vi "Cache.DUT.DataToTable.vi"(10 "Groups":i32[](array[numeric]), 11 "Results in":T1[](array[typedef])) -> (1 "Colors":u32[][](array[colorbox]), 2 "Headers":string[](array[string]), 3 "Values":string[][](array[string]))   [LabVIEW 2016]
uses:
  Database/Database.Global.vi
  Database/ProdaNG/Controls/ProdaNG.ProcessResult.ctl
  Database/ProdaNG/Controls/ProdaNG.ProcessStepResult.ctl
  Database/ProdaNG/Controls/ProdaNG.TestValueResult.ctl
  Database/ProdaNG/Controls/ProdaNG.TestStepResult.ctl
  Cache.TestSteps.Fglb.ResultData.ctl
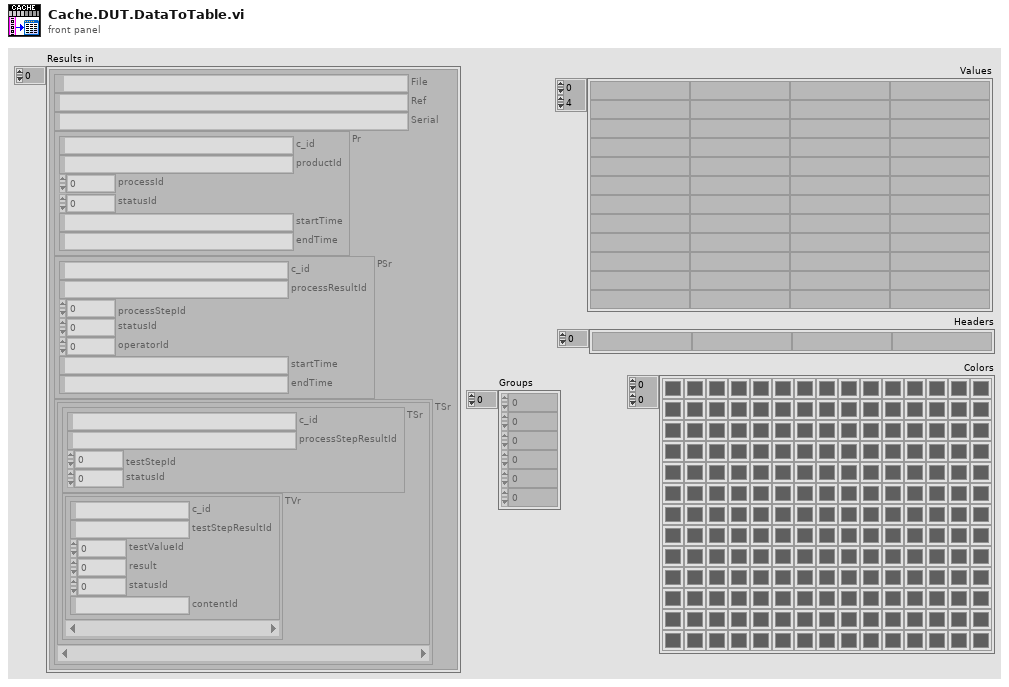
[diagram p1: front panel]
types:
  T1 = typedef "Cache.TestSteps.Fglb.ResultData.ctl" = cluster{"File":path, "Ref":string, "Serial":string, "Pr":T2, "PSr":T3, "TSr":cluster{"TSr":T4, "TVr":T5[]}[]}
  T2 = typedef "ProdaNG.ProcessResult.ctl" = cluster{"c_id":string, "productId":string, "processId":i32, "statusId":i32, "startTime":string, "endTime":string}
  T3 = typedef "ProdaNG.ProcessStepResult.ctl" = cluster{"c_id":string, "processResultId":string, "processStepId":i32, "statusId":i32, "operatorId":i32, "startTime":string, "endTime":string}
  T4 = typedef "ProdaNG.TestStepResult.ctl" = cluster{"c_id":string, "processStepResultId":string, "testStepId":i32, "statusId":i32}
  T5 = typedef "ProdaNG.TestValueResult.ctl" = cluster{"c_id":string, "testStepResultId":string, "testValueId":i32, "result":dbl, "statusId":i32, "contentId":string}
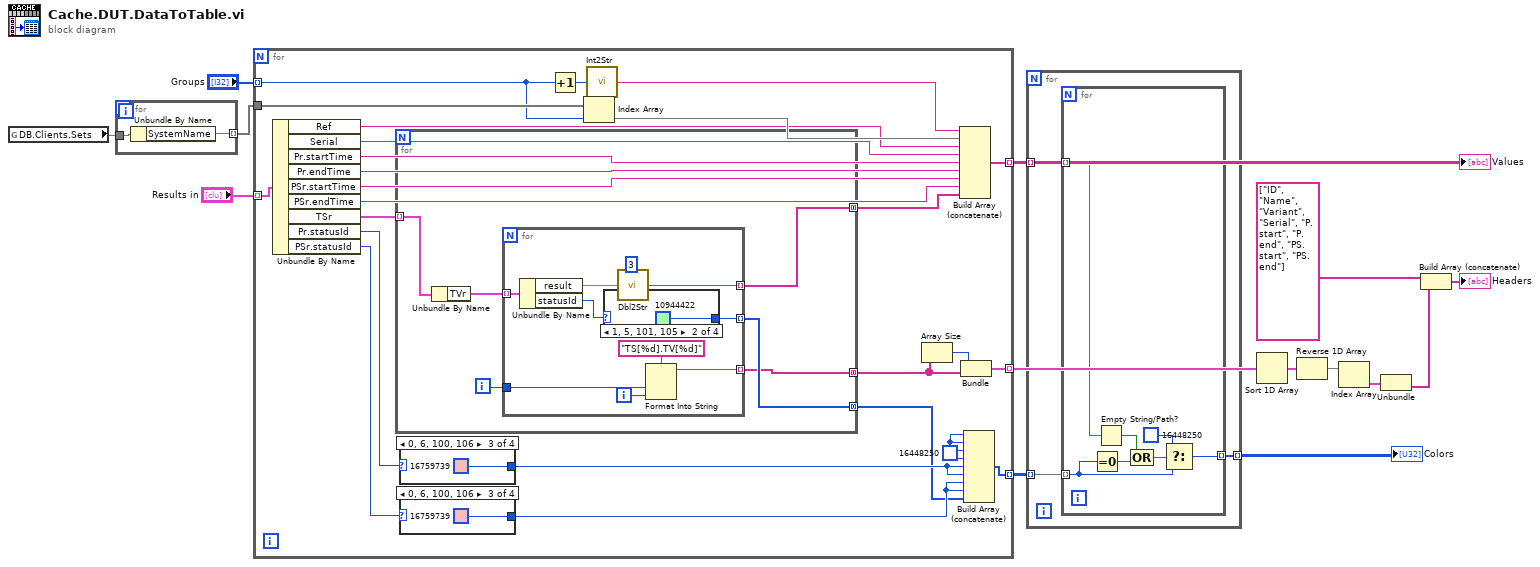
[diagram p0: block diagram]
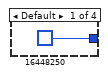
[diagram p2: hidden frame]
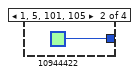
[diagram p3: hidden frame]
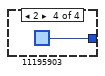
[diagram p4: hidden frame]
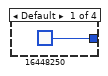
[diagram p5: hidden frame]
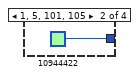
[diagram p6: hidden frame]
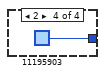
[diagram p7: hidden frame]
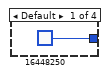
[diagram p8: hidden frame]
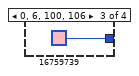
[diagram p9: hidden frame]
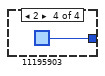
[diagram p10: hidden frame]
diagram:
  n1 = global read "Database.Global.vi" "DB.Clients.Sets"() -> (w10)
  n2 = for {
    tunnel: w10 -> [w16]
    tunnel: [w15] -> w1 mode=indexing
    n3 = Unbundle By Name(w16) -> ("SystemName"=w15)
  }
  n4 = for {
    tunnel: "Results in" -> [w41] mode=indexing
    tunnel: [w31] -> w12 mode=indexing
    tunnel: [w30] -> w13 mode=indexing
    tunnel: "Groups" -> [w21] mode=indexing
    tunnel: w1 -> [w27]
    tunnel: [w23] -> w9 mode=indexing
    w17 = u32 16448250
    n5 = Unbundle By Name(w41) -> ("Ref"=w19:string, "Serial"=w20:string, "Pr.startTime"=w40:string, "Pr.endTime"=w26:string, "PSr.startTime"=w39:string, "PSr.endTime"=w18:string, "TSr"=w38:cluster{"TSr":T4, "TVr":T5[]}[], "Pr.statusId"=w37:i32, "PSr.statusId"=w36:i32)
    n6 = for {
      tunnel: w38 -> [w55] mode=indexing
      tunnel: [w52] -> w33 mode=concatenating
      tunnel: [w51] -> w32 mode=concatenating
      tunnel: [w50] -> w24 mode=concatenating
      i -> [w53]
      n7 = Unbundle By Name(w55) -> ("TVr"=w54:T5[])
      n8 = for {
        tunnel: w54 -> [w65] mode=indexing
        tunnel: [w61] -> w52 mode=indexing
        tunnel: [w60] -> w51 mode=indexing
        tunnel: w53 -> [w57]
        tunnel: [w56] -> w50 mode=indexing
        i -> [w59]
        n9 = Unbundle By Name(w65) -> ("result"=w63:dbl, "statusId"=w64:i32)
        n10 = case shown="1, 5, 101, 105" w64 {
          tunnel: [u32 16448250 u32 10944422 u32 16759739 u32 11195903] -> w61
          frame Default {
          }
          frame 1, 5, 101, 105 {
          }
          frame 0, 6, 100, 106 {
          }
          frame 2 {
          }
        }
        n11 = call "Dbl2Str.vi"("Numeric"=w63, "precision (6)"=i16 3) -> ("string"=w60:string)
        n12 = Format Into String(format string="TS[%d].TV[%d]", w57, w59) -> (resulting string=w56:string)  [unwired: 2 in, 1 out]
      }
    }
    n13 = case shown="0, 6, 100, 106" w37 {
      tunnel: [u32 16448250 u32 10944422 u32 16759739 u32 11195903] -> w34
      frame Default {
      }
      frame 1, 5, 101, 105 {
      }
      frame 0, 6, 100, 106 {
      }
      frame 2 {
      }
    }
    n14 = case shown="0, 6, 100, 106" w36 {
      tunnel: [u32 16448250 u32 10944422 u32 16759739 u32 11195903] -> w35
      frame Default {
      }
      frame 1, 5, 101, 105 {
      }
      frame 0, 6, 100, 106 {
      }
      frame 2 {
      }
    }
    n15 = Increment(x=w21) -> (x+1=w28:i32)
    n16 = Index Array(array=w27, index=w21) -> (element=w25)
    n17 = call "Int2Str.vi"("Numeric"=w28) -> ("string"=w29:string)
    n18 = Array Size(array=w24) -> (size(s)=w22:i32)
    n19 = Build Array (concatenate)(w29, w25, w19, w20, w40, w26, w39, w18, w32) -> (w31:string[])
    n20 = Bundle(w22, w24) -> (w23:cluster{i32, string[]})  [unwired: 1 in]
    n21 = Build Array (concatenate)(w17, w17, w17, w17, w34, w34, w35, w35, w33) -> (w30:u32[])
  }
  "Values" <- w12
  n22 = for {
    tunnel: w12 -> [w71] mode=indexing
    tunnel: w13 -> [w72] mode=indexing
    tunnel: [w70] -> w6 mode=indexing
    n23 = for {
      tunnel: w72 -> [w75] mode=indexing
      tunnel: w71 -> [w79] mode=indexing
      tunnel: [w73] -> w70 mode=indexing
      n24 = Equal To 0?(x=w75) -> (x = 0?=w77:bool)
      n25 = Empty String/Path?(string/path=w79) -> (empty?=w78:bool)
      n26 = Compound Arithmetic op=OR(w78, w77) -> (w76:bool)
      n27 = Select(t=u32 16448250, s=w76, f=w75) -> (s? t:f=w73:u32)
    }
  }
  "Colors" <- w6
  n28 = Sort 1D Array(array=w9) -> (sorted array=w8:cluster{i32, string[]}[])
  n29 = Reverse 1D Array(array=w8) -> (reversed array=w7:cluster{i32, string[]}[])
  n30 = Index Array(array=w7) -> (element=w5:cluster{i32, string[]})  [unwired: 1 in]
  n31 = Unbundle(w5) -> (w4:string[])  [unwired: 1 out]
  n32 = Build Array (concatenate)(string[] ["ID", "Name", "Variant", "Serial", "P.start", "P.end", "PS.start", "PS.end"], w4) -> (→"Headers":string[])
